vi "cv_Labiew.vi"(0 "T [K]":dbl, 1 "1. Befüllschritt":u16(ring) items=["H2", "CH4", "C2H2", "O2", "N2"], 2 "2. Befüllschritt":u16(ring) items=["H2", "CH4", "C2H2", "O2", "N2"], 3 "3. Befüllschritt":u16(ring) items=["H2", "CH4", "C2H2", "O2", "N2"], 5 "Stoffmengenverhältnisse Vorbereitungsgase":dbl[](array[numeric]), 7 "Brenndauer":dbl, 9 "Aktuelle Zeit":dbl, 11 "Stoffmengenverhältnisse Gase nach 1. Verbrennung":dbl[](array[numeric]), 12 "4. Befüllschritt":u16(ring) items=["H2", "CH4", "C2H2", "O2", "N2"], 13 "5. Befüllschritt":u16(ring) items=["H2", "CH4", "C2H2", "O2", "N2"]) -> (4 "cv":dbl)   [LabVIEW 2009]
panel:
  in  "Koeffizienten der Gase":cluster{"Koeffizienten":dbl[]}[](array[cluster])
  # "H2"
  # "N2"
  # "CH4"
  # "O2"
  # "H2"
  # "C2H2"
  # "CH4"
  # "O2"
  # "C2H2"
  # "N2"
  # "CO2"
  # "CO2"
  # "H2O"
  # "H2O"
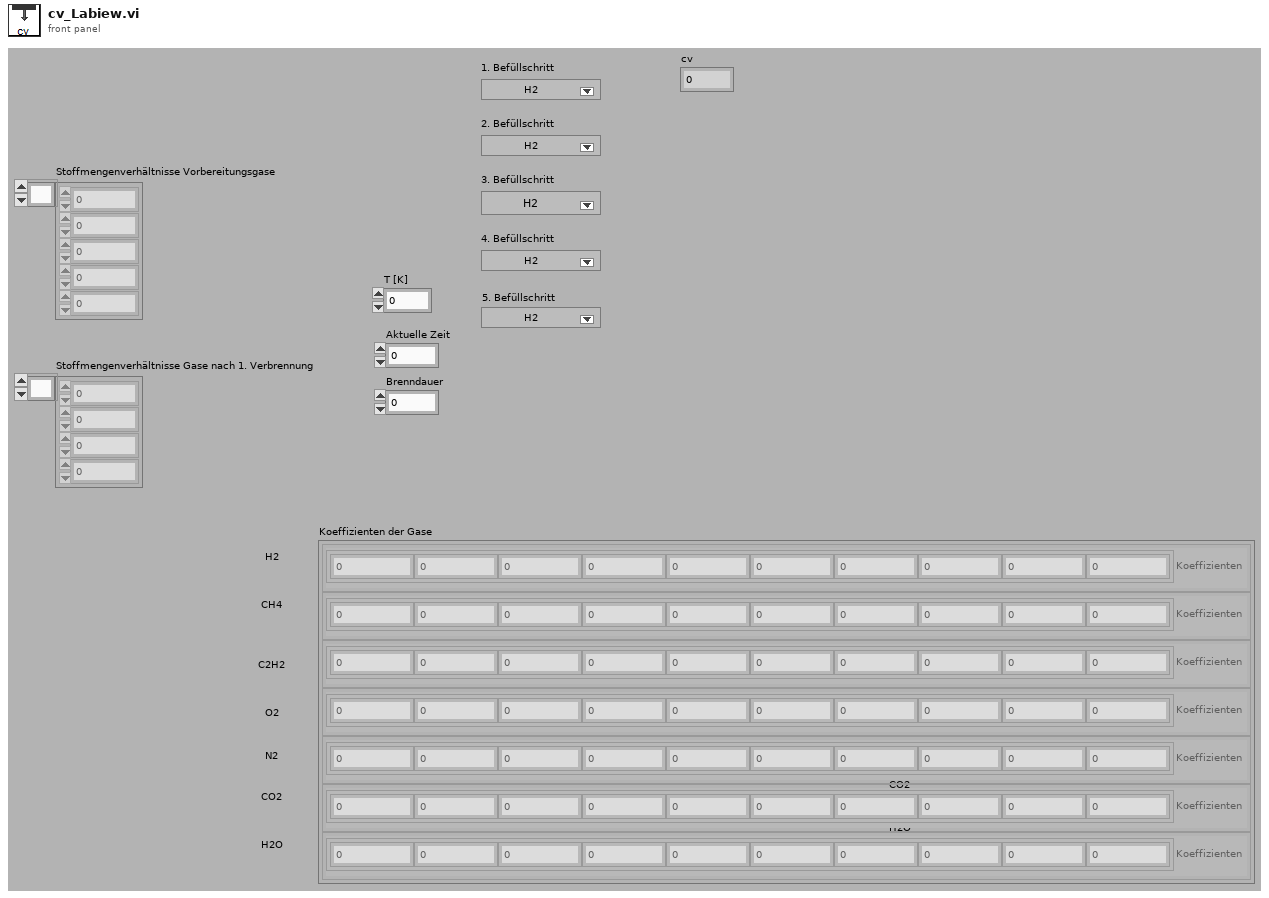
[diagram p1: front panel]
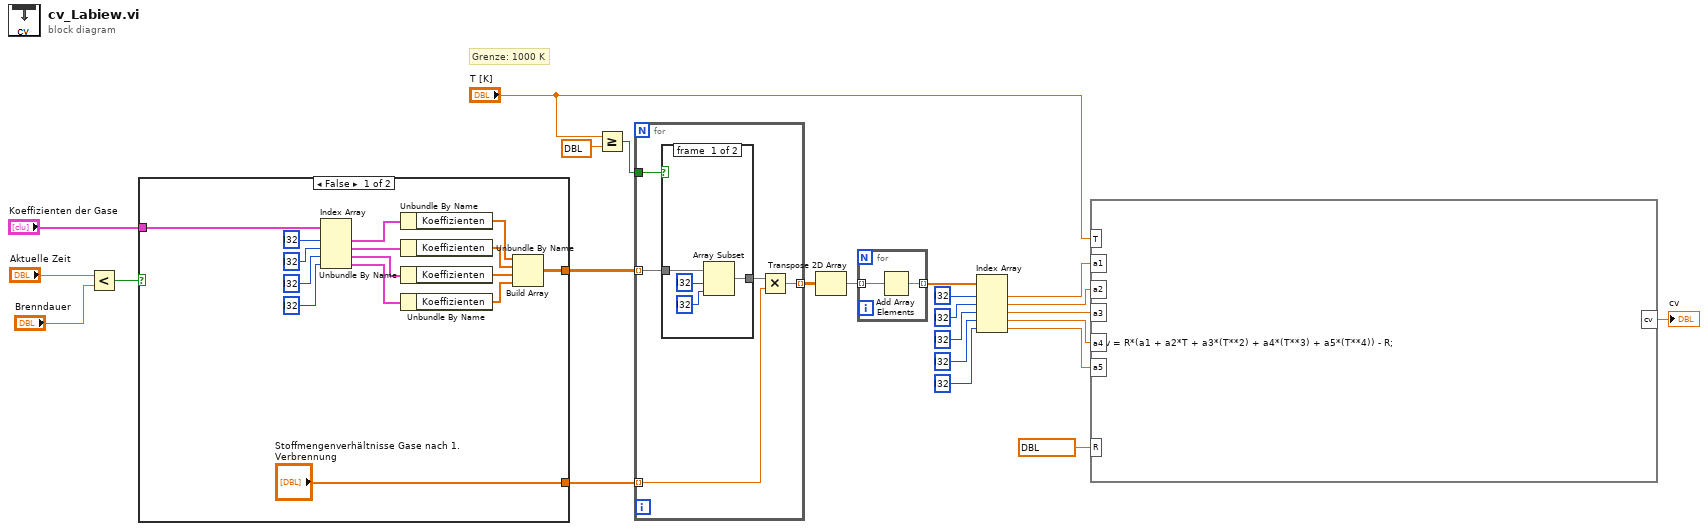
[diagram p0: block diagram]
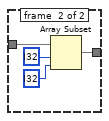
[diagram p2: hidden frame]
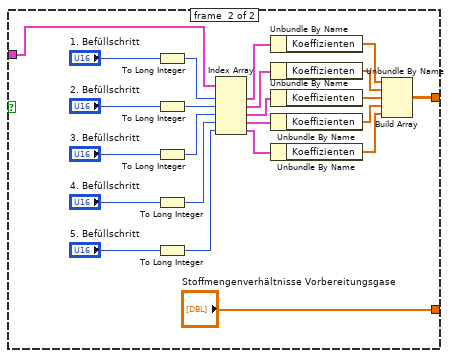
[diagram p3: hidden frame]
diagram:
  # "Grenze: 1000 K"
  n1 = Less?(x="Aktuelle Zeit", y="Brenndauer") -> (x < y?=w22:bool)
  n2 = case shown="False" w22 {
    tunnel: "Koeffizienten der Gase" -> [w39 w42]
    tunnel: ["Stoffmengenverhältnisse Gase nach 1. Verbrennung" "Stoffmengenverhältnisse Vorbereitungsgase"] -> w3
    tunnel: [w26 w40] -> w2
    frame #0 {
      n3 = Index Array(array=w39, index #1=i32 ? ("Index"), index #2=i32 ? ("Index"), index #3=i32 ? ("Index"), index #4=i32 ? ("Index")) -> (element #1=w34:cluster{"Koeffizienten":dbl[]}, element #2=w33:cluster{"Koeffizienten":dbl[]}, element #3=w32:cluster{"Koeffizienten":dbl[]}, element #4=w31:cluster{"Koeffizienten":dbl[]})
      n4 = Unbundle By Name(w34) -> ("Koeffizienten"=w27:dbl[])
      n5 = Unbundle By Name(w33) -> ("Koeffizienten"=w28:dbl[])
      n6 = Unbundle By Name(w32) -> ("Koeffizienten"=w29:dbl[])
      n7 = Unbundle By Name(w31) -> ("Koeffizienten"=w30:dbl[])
      n8 = Build Array(w27, w28, w29, w30) -> (w26:dbl[][])
    }
    frame #1 {
      n9 = To Long Integer(number="1. Befüllschritt") -> (32bit integer=w47:i32)
      n10 = To Long Integer(number="2. Befüllschritt") -> (32bit integer=w46:i32)
      n11 = To Long Integer(number="3. Befüllschritt") -> (32bit integer=w45:i32)
      n12 = To Long Integer(number="4. Befüllschritt") -> (32bit integer=w44:i32)
      n13 = To Long Integer(number="5. Befüllschritt") -> (32bit integer=w43:i32)
      n14 = Index Array(array=w42, index #1=w47, index #2=w46, index #3=w45, index #4=w44, index #5=w43) -> (element #1=w57:cluster{"Koeffizienten":dbl[]}, element #2=w56:cluster{"Koeffizienten":dbl[]}, element #3=w55:cluster{"Koeffizienten":dbl[]}, element #4=w54:cluster{"Koeffizienten":dbl[]}, element #5=w53:cluster{"Koeffizienten":dbl[]})
      n15 = Unbundle By Name(w57) -> ("Koeffizienten"=w52:dbl[])
      n16 = Unbundle By Name(w56) -> ("Koeffizienten"=w51:dbl[])
      n17 = Unbundle By Name(w55) -> ("Koeffizienten"=w50:dbl[])
      n18 = Unbundle By Name(w54) -> ("Koeffizienten"=w49:dbl[])
      n19 = Unbundle By Name(w53) -> ("Koeffizienten"=w48:dbl[])
      n20 = Build Array(w52, w51, w50, w49, w48) -> (w40:dbl[][])
    }
  }
  n21 = Greater Or Equal?(x="T [K]", y=dbl ?) -> (x >= y?=w5:bool)
  n22 = for {
    tunnel: w2 -> [w66] mode=indexing
    tunnel: w3 -> [w65] mode=indexing
    tunnel: w5 -> [w67]
    tunnel: [w63] -> w6 mode=indexing
    n23 = case shown="True" w67 {
      tunnel: w66 -> [w69 w73]
      tunnel: [w68 w72] -> w64
      frame #0 {
        n24 = Array Subset(array=w69, index=i32 ? ("Index"), length=i32 ? ("Länge")) -> (w68:dbl[])
      }
      frame #1 {
        n25 = Array Subset(array=w73, index=i32 ? ("Index"), length=i32 ? ("Länge")) -> (w72:dbl[])
      }
    }
    n26 = Multiply(x=w64, y=w65) -> (x*y=w63:dbl[])
  }
  n27 = Transpose 2D Array(2D array=w6) -> (transposed array=w7:dbl[][])
  n28 = for {
    tunnel: w7 -> [w77] mode=indexing
    tunnel: [w76] -> w8 mode=indexing
    n29 = Add Array Elements(numeric array=w77) -> (sum=w76:dbl)
  }
  n30 = Index Array(array=w8, index #1=i32 ? ("Index"), index #2=i32 ? ("Index"), index #3=i32 ? ("Index"), index #4=i32 ? ("Index"), index #5=i32 ? ("Index")) -> (element #1=w15:dbl, element #2=w16:dbl, element #3=w17:dbl, element #4=w18:dbl, element #5=w19:dbl)
  n31 = formula code="cv = R*(a1 + a2*T + a3*(T**2) + a4*(T**3) + a5*(T**4)) - R;"("a1"=w15, "a2"=w16, "a3"=w17, "a4"=w18, "a5"=w19, "R"=dbl ? ("Eingangsvariable"), "T"="T [K]") -> ("cv"=→"cv":dbl)
